vi "GCS3 End Block.vi"(0 "Line to Parse":string, 5 "error in":errorcluster, 6 "Expected GCS 3.0 Block Name":string) -> (14 "GCS 3.0 Block Name":string, 16 "Is GCS 3.0 Block?":bool, 19 "error out":errorcluster)   [LabVIEW 2020]
uses:
  Match Regular Expression.xnode
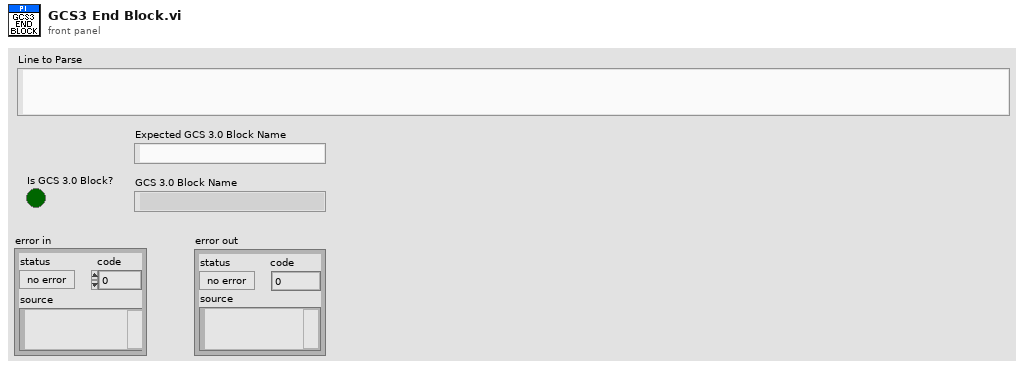
[diagram p1: front panel]
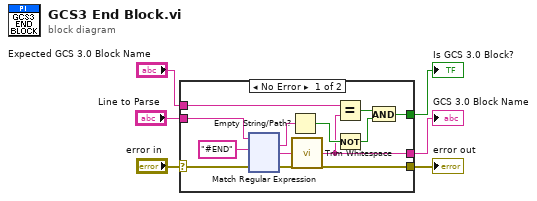
[diagram p0: block diagram]
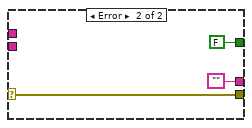
[diagram p2: hidden frame]
diagram:
  n1 = case shown="No Error" "error in" {
    selector: "error in" -> [w16 w135]
    tunnel: [w15 w135] -> w5
    tunnel: "Line to Parse" -> [w17 _]
    tunnel: [w7 FALSE] -> w3
    tunnel: [w11 ""] -> w2
    tunnel: "Expected GCS 3.0 Block Name" -> [w10 _]
    frame No Error {
      n2 = xnode "Match Regular Expression"("input string"=w17, "regular expression"="#END", "error in"=w16) -> ("whole match"=w14:string, "after match"=w12:string, "error out"=w15:errorcluster)  [unwired: 3 in, 2 out]
      n3 = Empty String/Path?(string/path=w14) -> (empty?=w13:bool)
      n4 = call "Trim Whitespace.vi"("string"=w12) -> ("trimmed string"=w11:string)  [unwired: 1 in]
      n5 = Equal?(x=w10, y=w11) -> (x = y?=w9:bool)
      n6 = Not(x=w13) -> (.not. x?=w8:bool)
      n7 = And(x=w9, y=w8) -> (x .and. y?=w7:bool)
    }
    frame Error {
    }
  }
  "error out" <- w5
  "Is GCS 3.0 Block?" <- w3
  "GCS 3.0 Block Name" <- w2
